vi "Offset.vi"(0 "Length T/2":i32=50, 1 "Offset":bool=TRUE, 2 "Pulse signal in":dbl[](array[numeric])) -> (6 "Pulse signal out":dbl[](array[numeric]))   [LabVIEW 2018]
panel:
  out "Pulse signal in graph out":dbl[](graph)
  out "Pulse signal in graph":dbl[](graph)
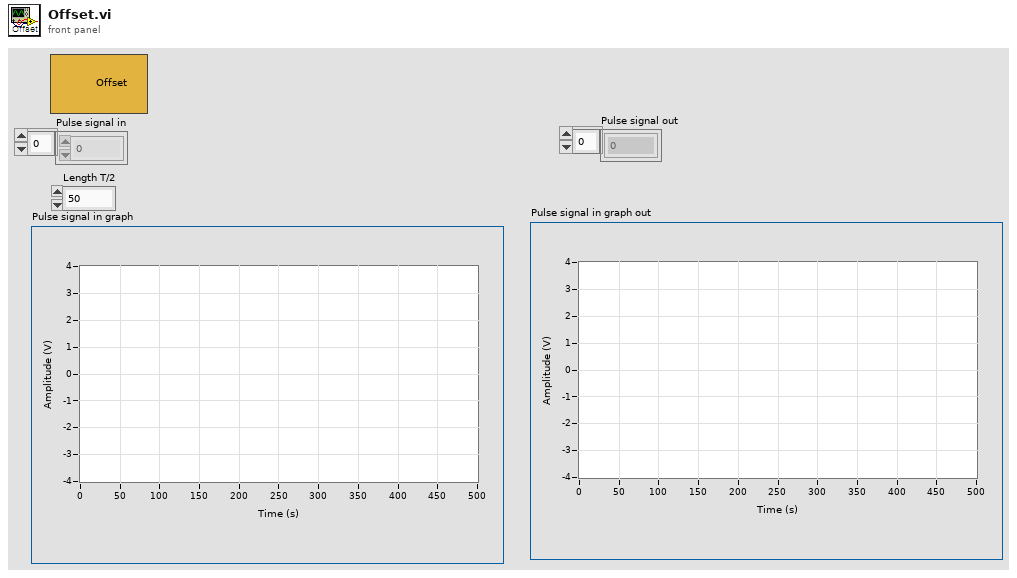
[diagram p1: front panel]
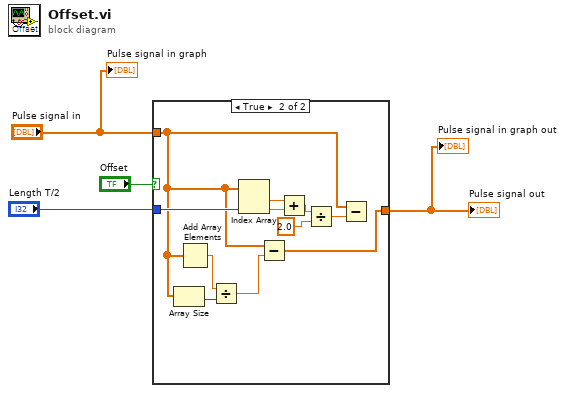
[diagram p0: block diagram]
diagram:
  n1 = case shown="True" "Offset" {
    tunnel: "Length T/2" -> [_ w14]
    tunnel: "Pulse signal in" -> [w5 w9]
    tunnel: [w5 w10] -> w2
    frame False {
    }
    frame True {
      n2 = Array Size(array=w9) -> (size(s)=w8:i32)
      n3 = Add Array Elements(numeric array=w9) -> (sum=w7:dbl)
      n4 = Divide(x=w7, y=w8) -> (x/y=w6:dbl)
      n5 = Index Array(array=w9, index #2=w14) -> (element #1=w12:dbl, element #2=w16:dbl)  [unwired: 1 in]
      n6 = Subtract(x=w9, y=w6) -> (x-y=w10:dbl[])
      n7 = Add(x=w12, y=w16) -> (x+y=w15:dbl)
      n8 = Divide(x=w15, y=2.0) -> (x/y=w11:dbl)
      n9 = Subtract(x=w9, y=w11) -> ()  [unwired: 1 out]
    }
  }
  "Pulse signal out" <- w2
  "Pulse signal in graph out" <- w2
  "Pulse signal in graph" <- "Pulse signal in"
